vi "getFPGAReference.vi"(11 "FPGA in":refnum<class "FPGA.lvclass">) -> (2 "FPGAReference":refnum<k20>, 3 "FPGA out":refnum<class "FPGA.lvclass">)   [LabVIEW 2016, in "FPGA.lvclass"]
uses:
  FPGA.lvclass
  FPGA.lvclass/FPGA.ctl
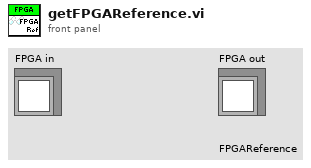
[diagram p1: front panel]
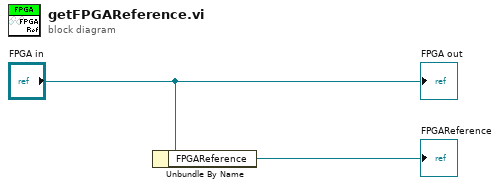
[diagram p0: block diagram]
diagram:
  n1 = Unbundle By Name("FPGA in") -> ("FPGAReference"=→"FPGAReference":refnum<k20>)
  "FPGA out" <- "FPGA in"
